vi "Topo & GridSpectr_DriftCorrection_v9.vi"(6 "Internal use":string, 7 "Grid param":T2 {"height (m)" format="%#_6p"; "width (m)" format="%#_6p"; "center Y (m)" format="%#_6p"; "center X (m)" format="%#_6p"}, 8 "Error in (no error)":errorcluster, 9 "Points Y/Index Y":i32, 10 "Points X/Index X":i32, 11 "Method":enum16{"init", "run", "end"}(ring)=enum."end") -> (0 "Error out":errorcluster)   [LabVIEW 2014]
doc: "Example of a measurement VI to be used in the \"Experiments on a Grid\" tool as external VI.\n\nThis example measure the topography and spectroscopy data. The spectroscopy measurements are taken on a subgrid. The data are saved to a sxm and a binary file.\n\n- Nanonis Programming Interface -"
uses:
  <userlib>/Nanonis Prog Interface V5/Nanonis Prog Interface.lvlib
  <userlib>/Nanonis Prog Interface V5/Scan/Grid/GridPatternGet.vi
panel:
  out "ETA":timestamp
  out "remaining":dbl
  out "Progress":u8(slide) scale=0.0..100.0 scale format="%#.1g"
  out "total Points":i32
  in  "preSTS delay [ms]":u32=3
  in  "STS Bias":dbl=0.005 format="%#_6p"
  in  "Move Bias":dbl=-0.01 format="%#_6p"
  in  "Move Current":dbl=1.5e-11 format="%#_6p"
  in  "Imaging Bias":dbl=-0.01 format="%#_6p"
  in  "max applied Drift Correction":i32=20 min=1 max=100 step=1 format="%.0p"
  in  "Correlate":u16(ring) items=["first Frame", "successive Frames"]
  out "Topo Images taken":i32=14
  in  "Increment":i32=40
  in  "Threshold":i32=2 min=1 step=1
  in  "tip Speed (m/s)":sgl=1e-08 format="%.2p"
  in  "Drift Correction 2":T1
  out "X drift":i32
  out "Y drift":i32
  out "Last Drift detected":i32=40
  in  "MaxImagesBack":i32=40
  in  "Channel index (0-23)":u8=14
  in  "File name":string="single_mol_shortSTS"
  in  "STS Current":dbl=1.15e-09 format="%#_6p"
  in  "Imaging Current":dbl=1.5e-11 format="%#_6p"
  in  "zdrift \nDuration (s)":dbl
  in  "Correct z drift":bool
  out "Status":string="finishing"
  in  "Drift correction Pixels":i32=256 caption="Topo Pixels"
  out "Y Offset":dbl format="%#_6p"
  out "X Offset":dbl format="%#_6p"
  out "Points taken":dbl=14.0
  in  "Drift Correction every":i32=40
  in  "Y subgrid spacing":u16=1
  in  "X subgrid spacing":u16=1
  # "GRID points"
  # "Increase this if no Drift was detected for \na certain number of images"
  # "images back"
  # "% of image size"
  # "RUN smart tilt before starting the GRID"
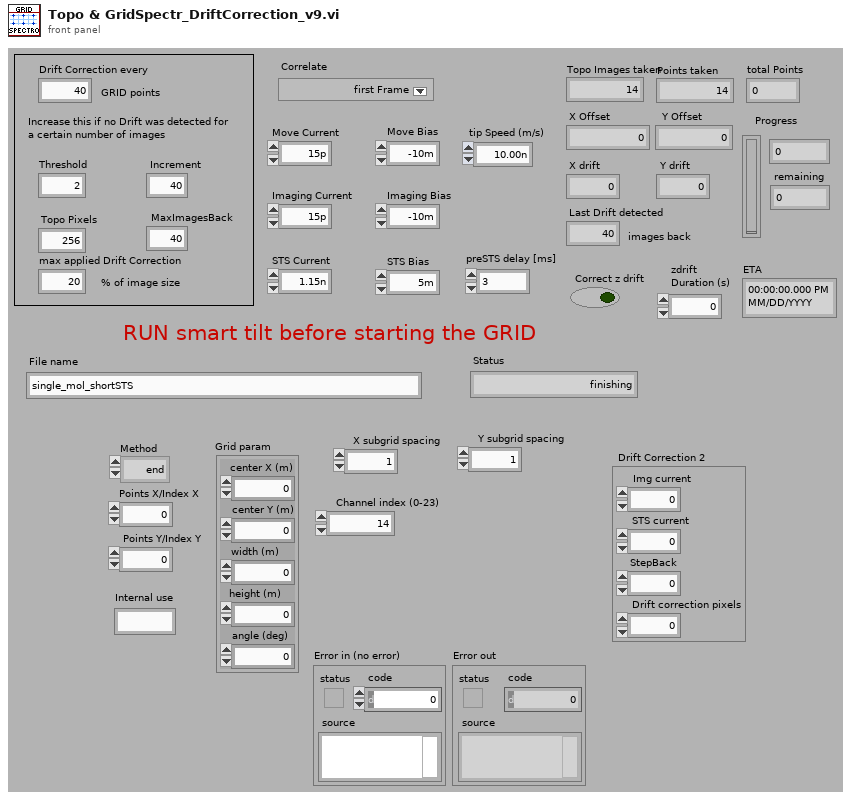
[diagram p1: front panel]
types:
  T1 = cluster{"Img current":dbl, "STS current":dbl, "StepBack":dbl, "Drift correction pixels":dbl}
  T2 = cluster{"center X (m)":sgl, "center Y (m)":sgl, "width (m)":sgl, "height (m)":sgl, "angle (deg)":sgl}
  T3 = cluster{"center X":sgl, "center Y":sgl, "angle":sgl, "width":sgl, "height":sgl, "# pixels":i32, "# lines":i32}
  T4 = cluster{"Name":string, "Calibration":sgl, "Offset":sgl, "Channel index":i32}[]
  T5 = cluster{"up/down":bool, "time/line":sgl, "start time":timestamp, "end time":timestamp}
  T6 = cluster{"Z averaging time (s)":sgl, "Z offset (m)":sgl, "Initial settling time (s)":sgl}
  T7 = cluster{"Max. slew rate (V/s)":sgl, "Settling time (s)":sgl, "Integration time (s)":sgl}
  T8 = cluster{"End settling time (s)":sgl, "Z control time (s)":sgl}
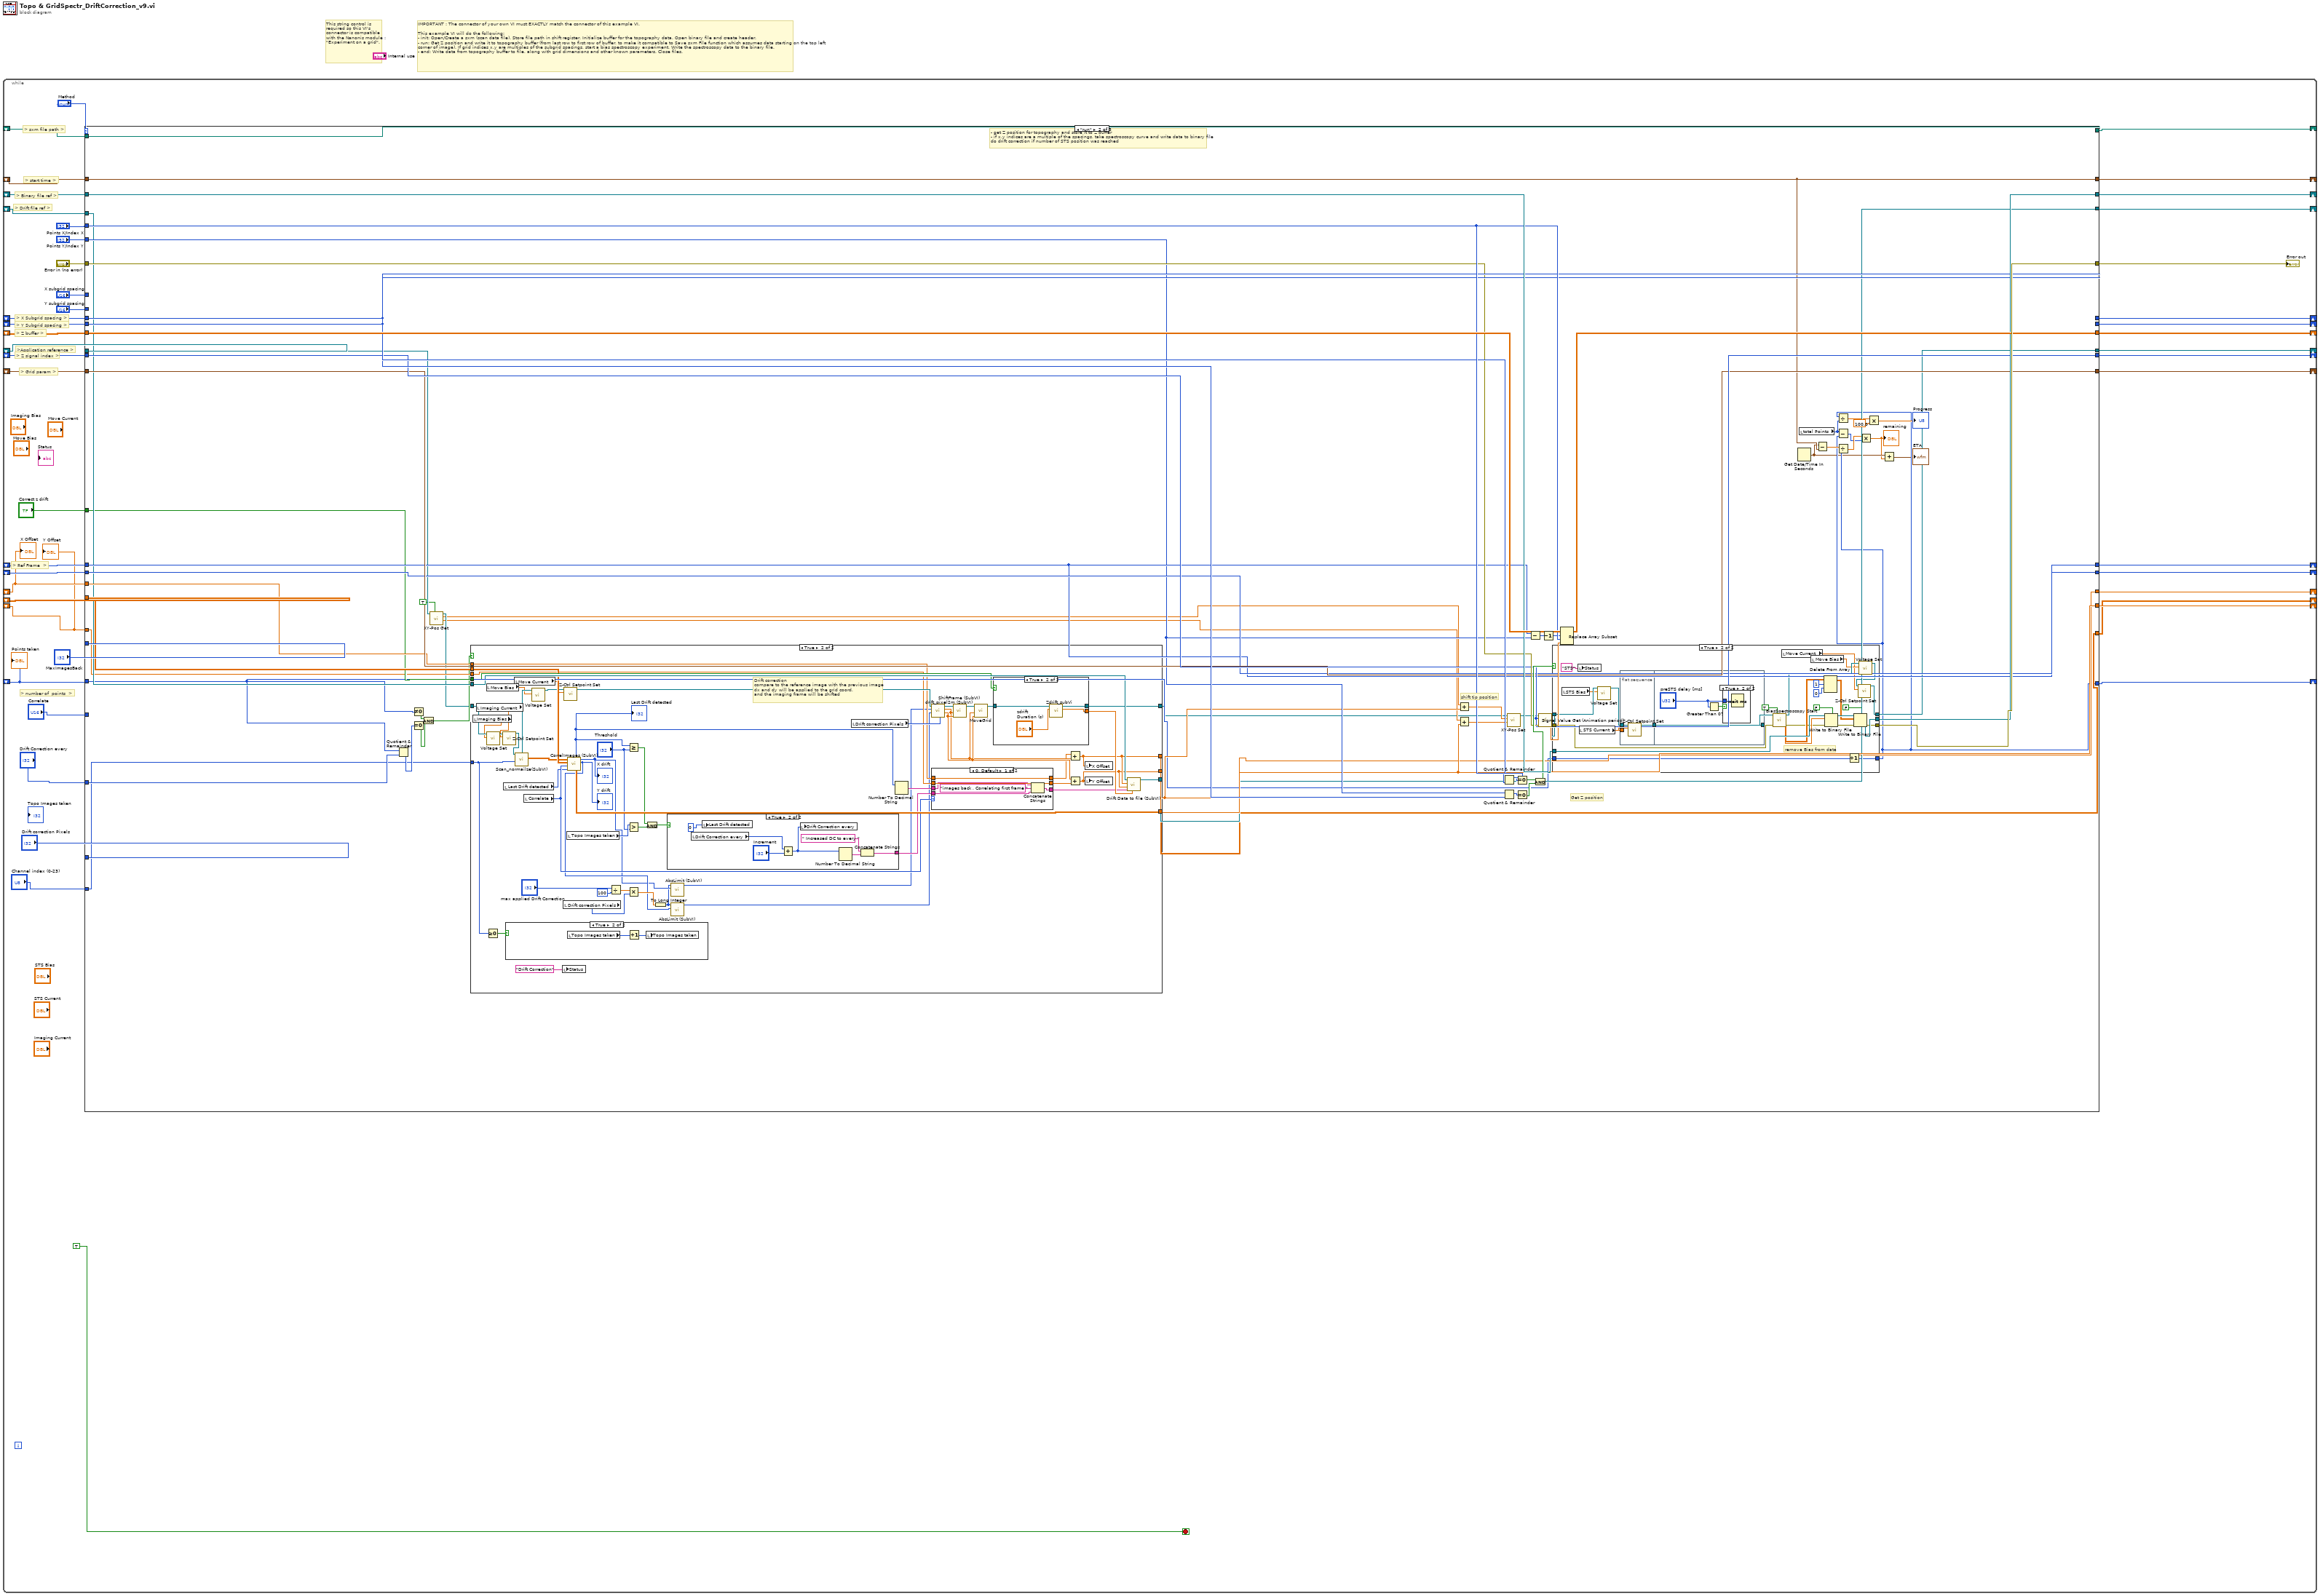
[diagram p0: block diagram]
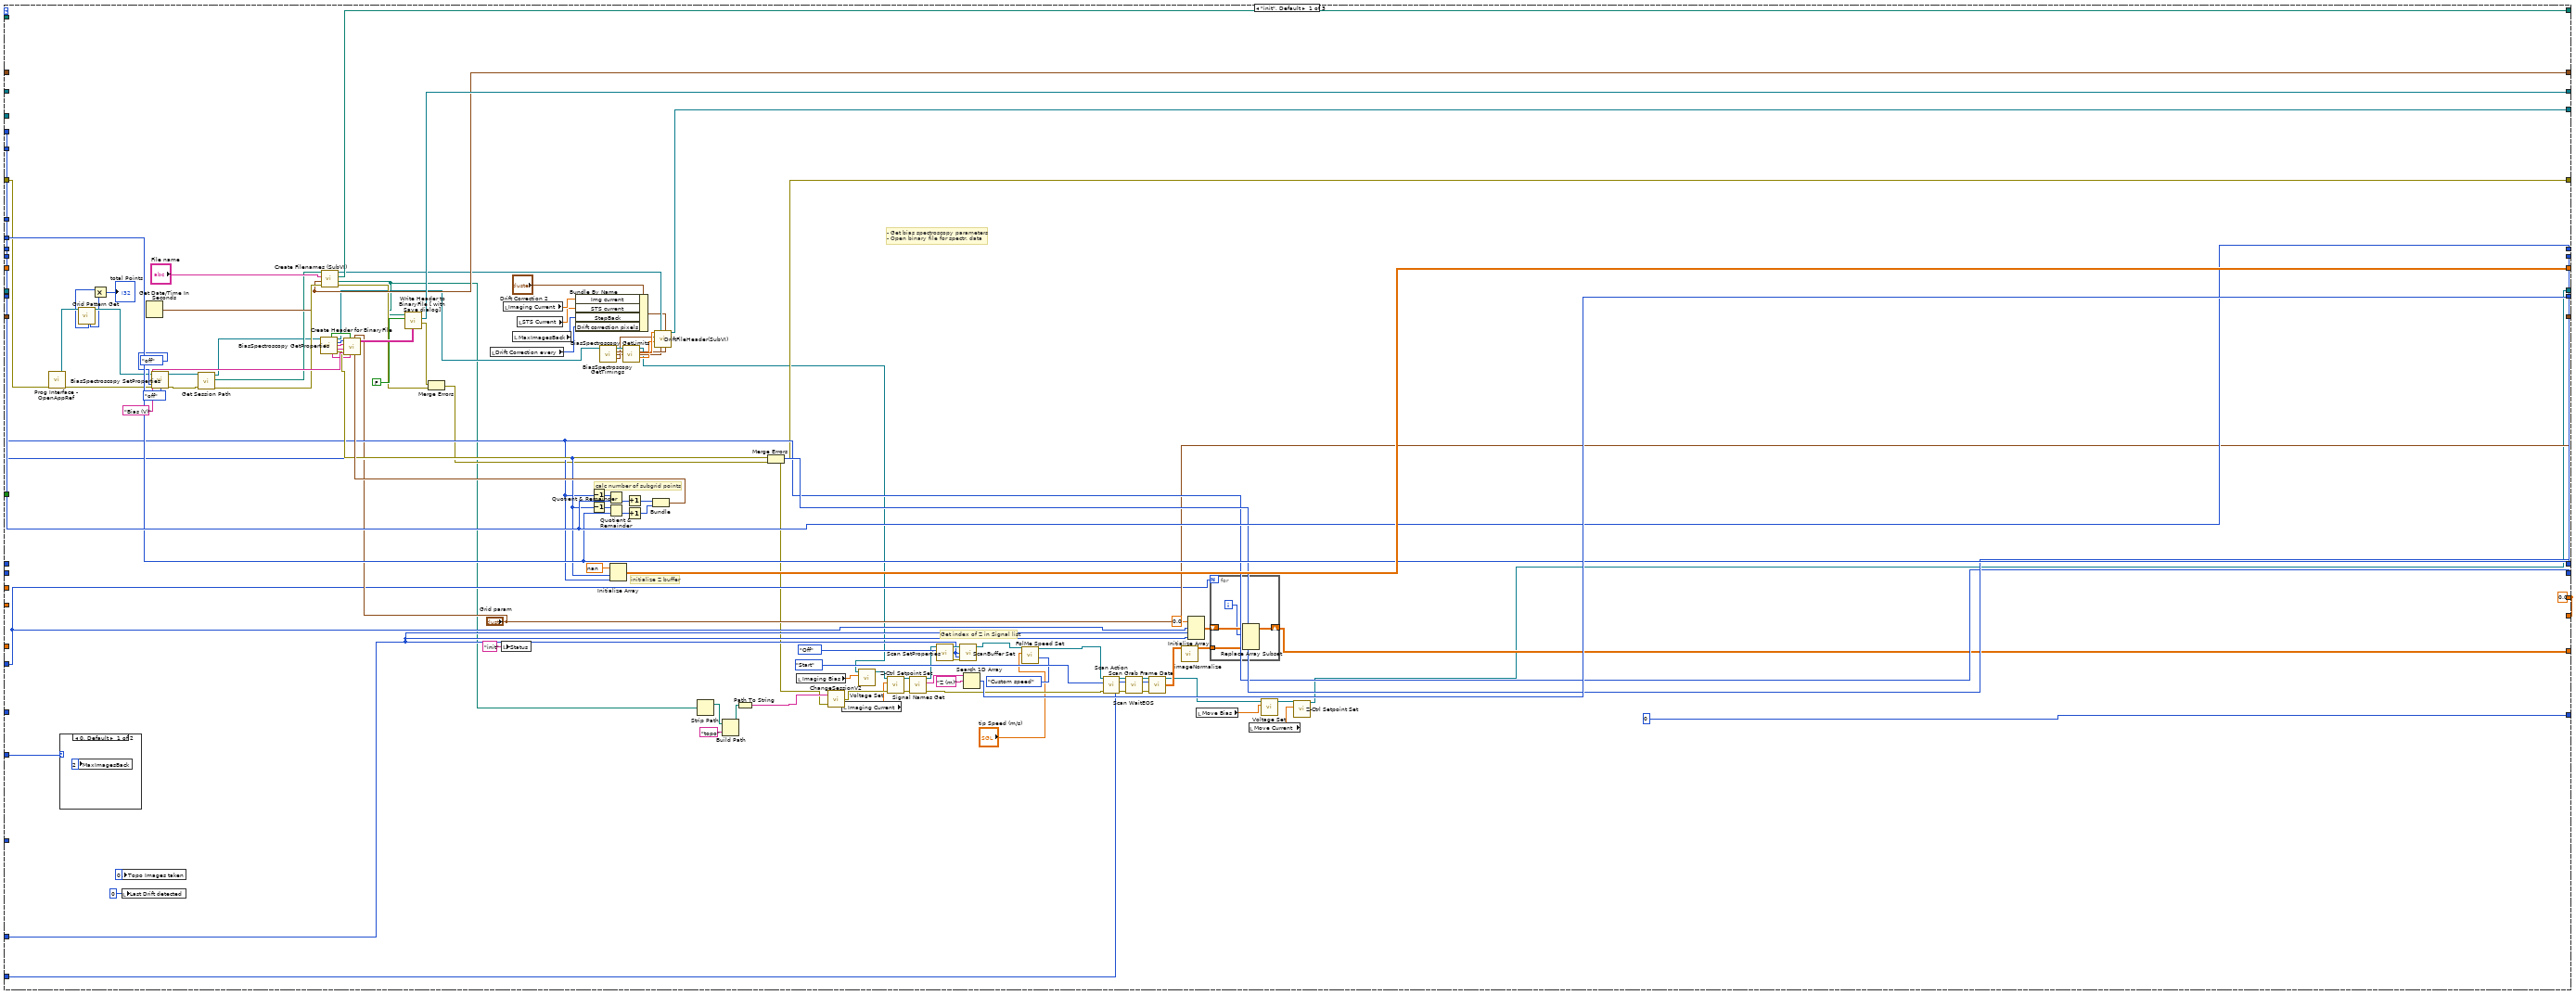
[diagram p2: hidden frame]
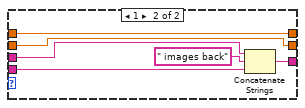
[diagram p5: hidden frame]
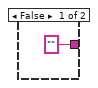
[diagram p7: hidden frame]
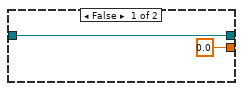
[diagram p8: hidden frame]
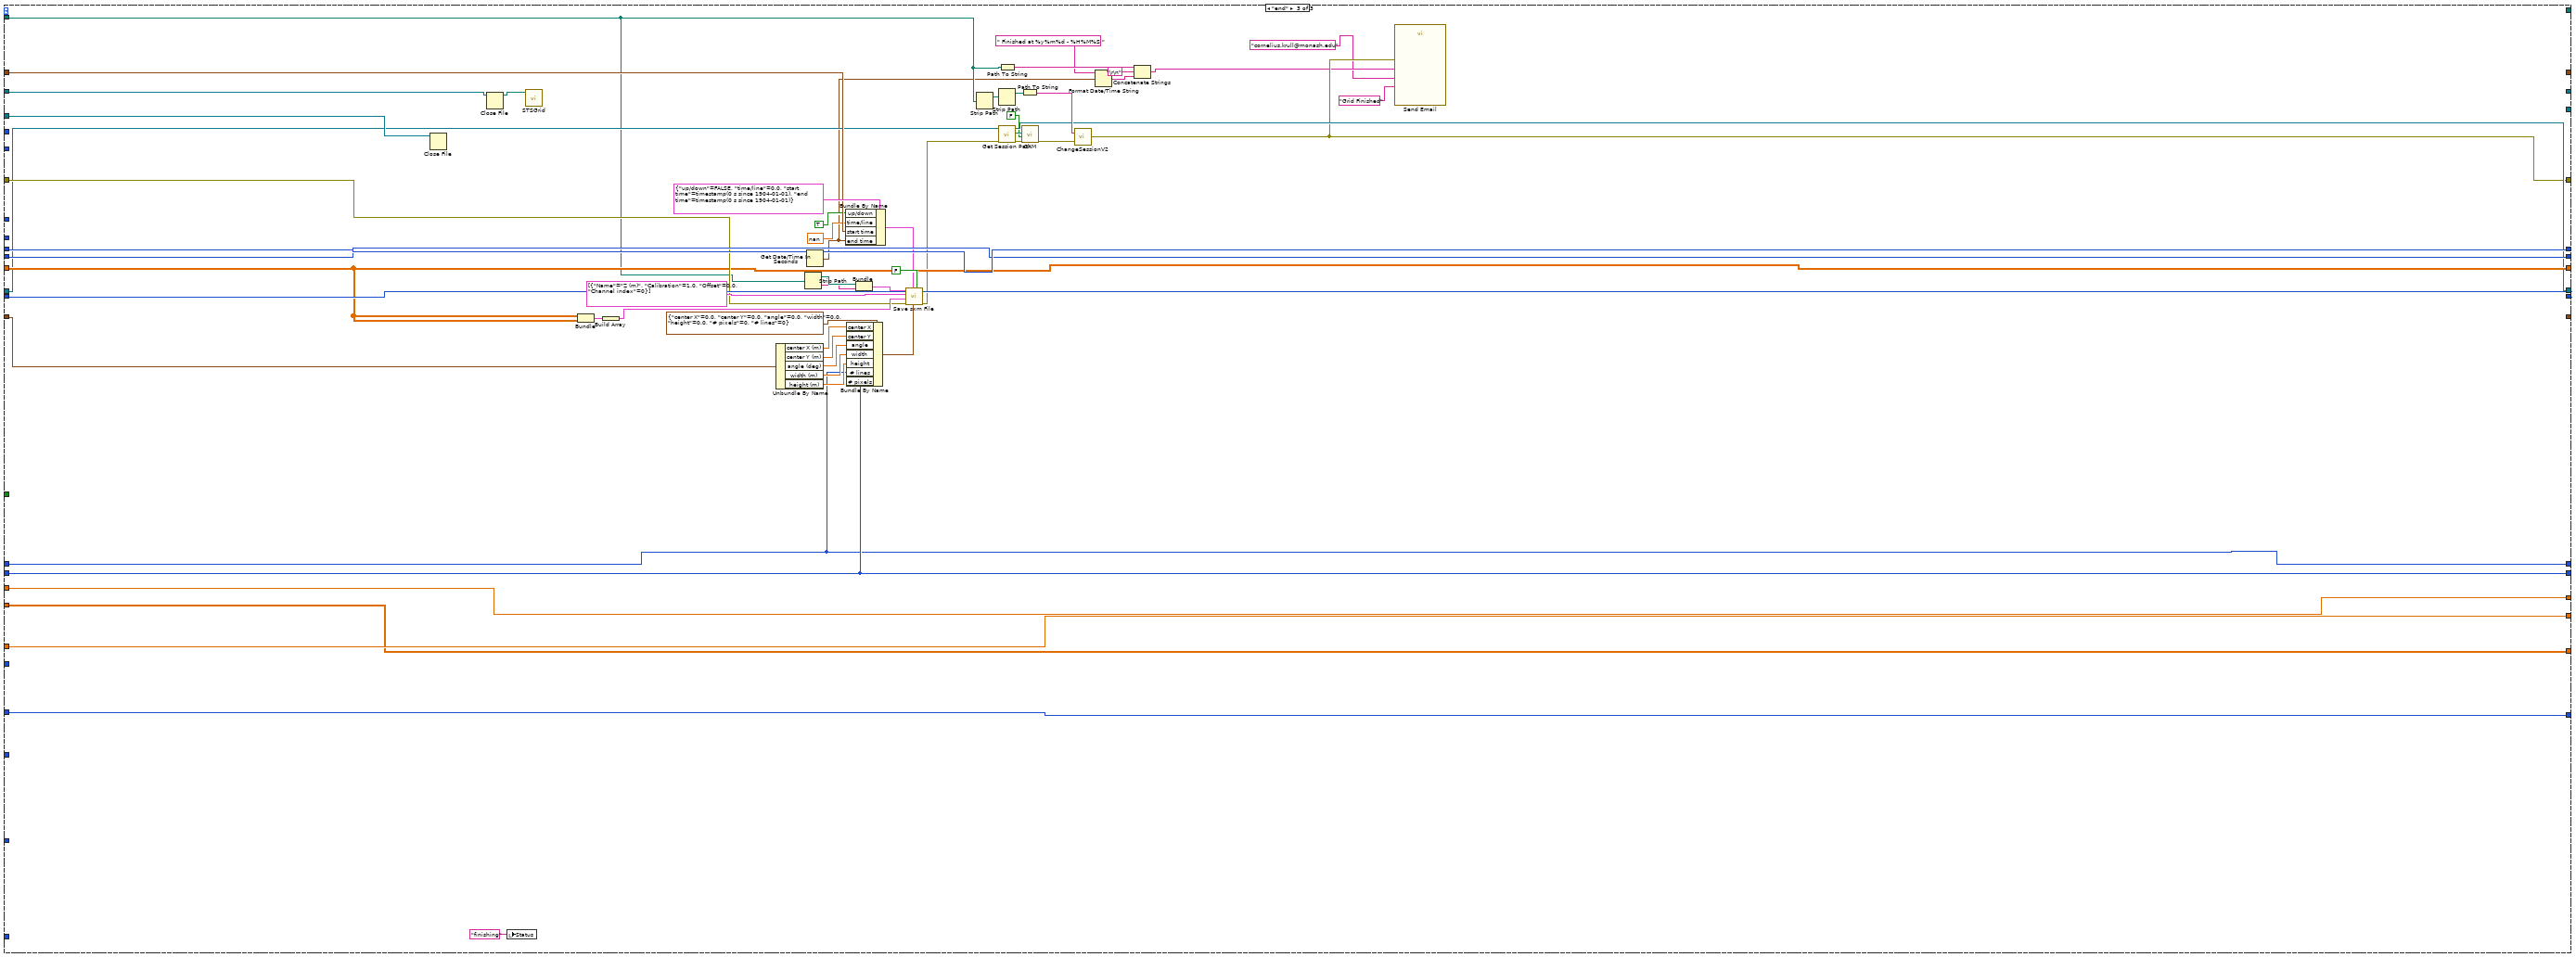
[diagram p11: hidden frame]
diagram:
  # "This string control is required so this VI's connector is compatible with the Nanonis module : \"Experiment on a grid\"."
  # "IMPORTANT : The connector of your own VI must EXACTLY match the connector of this example VI.\n\nThis example VI will do the following:\n- init: Open/Create a sxm (scan data file). Store file path in shift register. Initialize buffer for the topography data. Open binary file and create header.\n- run: Get Z position and write it to topography buffer (from last row to first row of buffer, to make it compatible to Save sxm File function which assumes data starting on the top left corner of image). If grid indices x,y are multiples of the subgrid spacings, start a bias spectroscopy experiment. Write the spectroscopy data to the binary file.\n- end: Write data from topography buffer to file, along with grid dimensions and other known parameters. Close files."
  n1 = while {
    shift-right: [w21] -> _
    shift-left: _ -> [w44]
    shift-right: [w39] -> _
    shift-left: _ -> [w38]
    shift-right: [w36] -> _
    shift-left: _ -> [w37]
    shift-right: [w35] -> _
    shift-left: _ -> [w34]
    shift-right: [w28] -> _
    shift-left: _ -> [w30]
    shift-right: [w29] -> _
    shift-left: _ -> [w31]
    shift-right: [w27] -> _
    shift-left: _ -> [w26]
    shift-right: [w25] -> _
    shift-left: _ -> [w24]
    shift-right: [w23] -> _
    shift-left: _ -> [w22]
    shift-right: [w20] -> _
    shift-left: _ -> [w19]
    shift-right: [w18] -> _
    shift-left: _ -> [w17]
    shift-right: [w16] -> _
    shift-left: _ -> [w9]
    shift-right: [w15] -> _
    shift-left: _ -> [w8]
    shift-right: [w14] -> _
    shift-left: _ -> [w11]
    shift-right: [w13] -> _
    shift-left: _ -> [w10]
    shift-right: [w6] -> _
    shift-left: _ -> [w5]
    stop <- TRUE stop-if-true
    # "> Drift file ref >"
    # "> number of  points  >"
    # "> Ref Frame  >"
    # "> Grid param >"
    # "> start time >"
    # ">Application reference >"
    # "> Y Subgrid spacing >"
    # "> X Subgrid spacing >"
    # "> Z signal index >"
    # "> Binary file ref >"
    # "> Z buffer >"
    # "> sxm file path >"
    n2 = case shown="\"run\"" "Method" {
      tunnel: [w109 w222 _] -> w21
      tunnel: w44 -> [_ w222 w358]
      tunnel: "Error in (no error)" -> [w111 w208 w390]
      tunnel: [w72 w221 w359] -> w42
      tunnel: "Points X/Index X" -> [w130 w216 _]
      tunnel: "Points Y/Index Y" -> [w131 w201 _]
      tunnel: [w154 w219 w379] -> w39
      tunnel: w38 -> [_ w220 w379]
      tunnel: w37 -> [_ w218 w372]
      tunnel: [w146 w217 _] -> w36
      tunnel: [w144 w206 w404] -> w35
      tunnel: w34 -> [_ w206 w404]
      tunnel: "X subgrid spacing" -> [w143 _ _]
      tunnel: "Y subgrid spacing" -> [w142 _ _]
      tunnel: w31 -> [_ w210 w403]
      tunnel: w30 -> [_ w209 w402]
      tunnel: [w143 w210 w403] -> w29
      tunnel: [w142 w209 w402] -> w28
      tunnel: [w60 w194 w364] -> w27
      tunnel: w26 -> [_ w177 w365]
      tunnel: ["Grid param" w204 _] -> w25
      tunnel: w24 -> [_ w204 w389]
      tunnel: [w108 w167 _] -> w23
      tunnel: w22 -> [_ w167 w397]
      tunnel: [w131 w202 w380] -> w20
      tunnel: w19 -> [_ w202 w380]
      tunnel: [w130 w203 w381] -> w18
      tunnel: w17 -> [_ w203 w381]
      tunnel: [w121 w184 w378] -> w16
      tunnel: [w121 w189 w376] -> w15
      tunnel: [w103 w183 w373] -> w14
      tunnel: [0 w165 w377] -> w13
      tunnel: w10 -> [_ w180 w377]
      tunnel: "Drift Correction every" -> [_ w197 _]
      tunnel: w11 -> [_ w188 w373]
      tunnel: w9 -> [_ w195 w378]
      tunnel: w8 -> [_ w181 w376]
      tunnel: "Drift correction Pixels" -> [w102 _ _]
      tunnel: [w98 w186 _] -> w6
      tunnel: w5 -> [_ w187 w374]
      tunnel: "Correct z drift" -> [_ w185 _]
      tunnel: "Channel index (0-23)" -> [w106 w182 _]
      tunnel: "MaxImagesBack" -> [w101 _ _]
      tunnel: "Correlate" -> [w63 _ _]
      frame "init", Default {
        w121 = 0.0
        # "- Get bias spectroscopy parameters\n- Open binary file for spectr. data"
        # "initialize Z buffer"
        # "calc number of subgrid points"
        # "Get index of Z in Signal list"
        n3 = call <userlib>:"Prog Interface - OpenAppRef.vi"("Error in (no error)"=w111) -> ("Error out"=w70:errorcluster, "Application reference"=w51:refnum<vi>)  [unwired: 5 in]
        n4 = case shown="0, Default" w63 {
          frame 0, Default {
            n5 = local write "MaxImagesBack"(2 ("StepsBack")) -> ()
          }
          frame 1 {
          }
        }
        n6 = call-poly <userlib>:"Grid Pattern Get.vi"("Application ref in"=w51) -> ("Points Y"=w48:i32, "Points X"=w49:i32, "Application ref out"=w50:refnum<vi>)  [unwired: 10 in, 6 out]
        n7 = Multiply(x=w48, y=w49) -> (x*y=→"total Points":i32)
        n8 = local write "Topo Images taken"(0 ("Images taken")) -> ()
        n9 = local write "Last Drift detected"(0 ("Last Drift detected")) -> ()
        n10 = Get Date/Time In Seconds() -> (seconds since 1Jan1904=w108:timestamp)
        n11 = call <userlib>:"BiasSpectroscopy SetProperties.vi"("Application ref in"=w50, "Autosave (no change)"=enum16{"no change", "on", "off"}."off", "Error in (no error)"=w70, "Save dialog"=enum16{"no change", "on", "off"}."off") -> ("Application ref out"=w66:refnum<vi>, "Error out"=w65:errorcluster)  [unwired: 10 in]
        n12 = call <userlib>:"Get Session Path.vi"("error in (no error)"=w65, "Application ref in"=w66) -> ("error out"=w110:errorcluster, "Session path"=w78:path, "Application ref out"=w67:refnum<vi>)  [unwired: 7 in]
        n13 = call <userlib>:"BiasSpectroscopy GetProperties.vi"("Application ref in"=w67) -> ("Backward sweep"=w150:bool, "Application ref out"=w82:refnum<vi>, "Number of points"=w133:i32, "Channels"=w132:string[], "Parameters"=w148:string[], "Fixed parameters"=w135:string[], "Error out"=w147:errorcluster)  [unwired: 6 in, 2 out]
        n14 = call "Create Filenames (SubVI).vi"("error in (no error)"=w110, "seconds since 1Jan1904"=w108, "File name"="File name", "Session path"=w78) -> ("error out"=w83:errorcluster, "binFilePath"=w74:path, "topoFilePath"=w109:path, "Drift File out"=w99:refnum<file>)  [unwired: 4 in]
        n15 = local read "Drift Correction every"() -> (w93:i32)
        n16 = local write "Status"("init" ("Status")) -> ()
        n17 = local read "Imaging Current"() -> (w95:dbl)
        n18 = local read "MaxImagesBack"() -> (w92:i32)
        n19 = local read "STS Current"() -> (w94:dbl)
        n20 = Bundle By Name(cluster="Drift Correction 2", "Img current"=w95, "STS current"=w94, "StepBack"=w92, "Drift correction pixels"=w93) -> (w96:T1)
        n21 = Decrement(x=w130) -> (x-1=w141:i32)
        n22 = Decrement(x=w131) -> (x-1=w140:i32)
        n23 = call <userlib>:"BiasSpectroscopy GetTimings.vi"("Application ref in"=w82) -> ("Application ref out"=w91:refnum<vi>, "Initialization"=w88:T6, "Sweep Timing"=w86:T7, "End of Sweep"=w87:T8)  [unwired: 10 in, 1 out]
        n24 = Quotient & Remainder(x=w141, y=w143) -> (floor(x/y)=w139:i32)  [unwired: 1 out]
        n25 = Quotient & Remainder(x=w140, y=w142) -> (floor(x/y)=w138:i32)  [unwired: 1 out]
        n26 = Initialize Array(sgl nan ("element"), w131, w130) -> (w154:sgl[][])
        n27 = call <userlib>:"BiasSpectroscopy GetLimits.vi"("Application ref in"=w91) -> ("End value (V)"=w89:sgl, "Start value (V)"=w90:sgl, "Application ref out"=w58:refnum<vi>)  [unwired: 5 in, 1 out]
        n28 = Increment(x=w139) -> (x+1=w137:i32)
        n29 = Increment(x=w138) -> (x+1=w136:i32)
        n30 = Bundle(w137, w136) -> (w149:cluster{i32, i32})  [unwired: 1 in]
        n31 = call <userlib>:"Create Header for BinaryFile.vi"("Grid points"=w149, "Grid param"="Grid param", "Fixed parameters"=w135, "Backward sweep"=w150, "Sweep signal"="Bias (V)" ("Sweep Signal"), "Parameters"=w148, "Channels"=w132, "Points per sweep"=w133) -> ("Header (fixed attributes)"=w152:string[][])  [unwired: 3 in]
        n32 = call <userlib>:"Write Header to BinaryFile [ with Save dialog].vi"("Fixed Attributes"=w152, "Show Dialog? (T)"=FALSE, "Filename"=w74) -> ("Error out"=w84:errorcluster, "File ref"=w146:refnum<file>)  [unwired: 5 in, 2 out]
        n33 = Merge Errors(w84, w83) -> (w85:errorcluster)
        n34 = call "DriftFileHeader(SubVI).vi"("Initialization"=w88, "Drift Correction"=w96, "Sweep Timing"=w86, "Byte Stream File in"=w99, "End value (V)"=w89, "End of Sweep"=w87, "Start value (V)"=w90) -> ("Byte Stream File out"=w98:refnum<file>)  [unwired: 4 in]
        n35 = Strip Path(path=w74) -> (stripped path=w77:path)  [unwired: 1 out]
        n36 = Build Path(base path=w77, name or relative path="topo") -> (appended path=w75:path)
        n37 = Path To String(path=w75) -> (string=w73:string)
        n38 = Merge Errors(w147, w85) -> (w72:errorcluster)
        n39 = local read "Imaging Bias"() -> (w54:dbl)
        n40 = call "ChangeSessionV2.vi"("error in (no error)"=w72, "Session"=w73) -> ("error out"=w71:errorcluster)
        n41 = local read "Imaging Current"() -> (w53:dbl)
        n42 = call <userlib>:"Voltage Set.vi"("Bias (V)"=w54, "Application ref in"=w58) -> ("Application ref out"=w57:refnum<vi>)  [unwired: 8 in, 1 out]
        n43 = call <userlib>:"Z-Ctrl Setpoint Set.vi"("error in (no error)"=w71, "Z Controller setpoint"=w53, "Application ref in"=w57) -> ("error out"=w112:errorcluster, "Application ref out"=w113:refnum<vi>)  [unwired: 7 in]
        n44 = call <userlib>:"Signal Names Get.vi"("error in (no error)"=w112, "Application ref in"=w113) -> ("error out"=w122:errorcluster, "Signals Names"=w134:string[], "Application ref out"=w117:refnum<vi>)  [unwired: 5 in]
        n45 = call <userlib>:"Scan SetProperties.vi"("Application ref in"=w117, "Continuous scan"=enum16{"No change", "On", "Off"}."Off") -> ("Application ref out"=w119:refnum<vi>, "Error out"=w118:errorcluster)  [unwired: 12 in]
        n46 = call <userlib>:"ScanBuffer Set.vi"("Application ref in"=w119, "Pixels"=w102, "Lines"=w102, "error in (no error)"=w118) -> ("Application ref out"=w61:refnum<vi>)  [unwired: 10 in, 1 out]
        n47 = Search 1D Array(1D array=w134, element="Z (m)") -> (index of element=w144:i32)  [unwired: 1 in]
        n48 = call <userlib>:"FolMe Speed Set.vi"("Speed Setting (Custom)"=enum32{"Scan speed", "Custom speed"}."Custom speed", "Speed (m/s)"="tip Speed (m/s)", "Application ref in"=w61) -> ("Application ref out"=w81:refnum<vi>)  [unwired: 5 in, 1 out]
        n49 = call <userlib>:"Scan Action.vi"("error in (no error)"=w122, "Scan action (Start)"=enum16{"Start", "Stop", "Pause", "Resume"}."Start", "Application ref in"=w81) -> ("error out"=w128:errorcluster, "Application ref out"=w127:refnum<vi>)  [unwired: 6 in]
        n50 = call <userlib>:"Scan WaitEOS.vi"("error in (no error)"=w128, "Application ref in"=w127) -> ("error out"=w125:errorcluster, "Application ref out"=w126:refnum<vi>)  [unwired: 5 in, 2 out]
        n51 = call <userlib>:"Scan Grab Frame Data.vi"("Application ref in"=w126, "Channel index (0-23)"=w106, "error in (no error)"=w125) -> ("Application ref out"=w52:refnum<vi>, "Scan frame data"=w114:sgl[][])  [unwired: 8 in, 3 out]
        n52 = call "imageNormalize.vi"("Data"=w114) -> ("Array"=w100:dbl[][])  [unwired: 10 in]
        n53 = Initialize Array(0.0 ("element"), w101, w102, w102) -> (w104:dbl[][][])
        n54 = local read "Move Bias"() -> (w56:dbl)
        n55 = for {
          N: w101 -> [_]
          tunnel: w100 -> [w158]
          shift-right: [w157] -> w103
          shift-left: w104 -> [w159]
          i -> [w156]
          n56 = Replace Array Subset(array=w159, new element=w158, index (dim 0)=w156) -> (w157:dbl[][][])  [unwired: 2 in]
        }
        n57 = local read "Move Current"() -> (w55:dbl)
        n58 = call <userlib>:"Voltage Set.vi"("Bias (V)"=w56, "Application ref in"=w52) -> ("Application ref out"=w59:refnum<vi>)  [unwired: 8 in, 1 out]
        n59 = call <userlib>:"Z-Ctrl Setpoint Set.vi"("Z Controller setpoint"=w55, "Application ref in"=w59) -> ("Application ref out"=w60:refnum<vi>)  [unwired: 8 in, 1 out]
      }
      frame "run" {
        # "shift tip position"
        # "Get Z position"
        # "- get Z position for topography and store it to Z buffer\n- if x,y indices are a multiple of the spacings, take spectroscopy curve and write data to binary file\ndo drift correction if number of STS position was reached"
        n60 = Quotient & Remainder(x=w180, y=w197) -> (x-y*floor(x/y)=w198:i32)  [unwired: 1 out]
        n61 = Not Equal To 0?(x=w180) -> (x != 0?=w178:bool)
        n62 = Equal To 0?(x=w198) -> (x = 0?=w196:bool)
        n63 = And(x=w178, y=w196) -> (x .and. y?=w179:bool)
        n64 = call <userlib>:"XY-Pos Get.vi"("Wait for newest data (F=False)"=TRUE, "Application ref in"=w177) -> ("Y (m)"=w173:sgl, "X (m)"=w174:sgl, "Application ref out"=w176:refnum<vi>)  [unwired: 5 in, 1 out]
        n65 = case shown="True" w179 {
          tunnel: w176 -> [w227 w235]
          tunnel: [w227 w277] -> w172
          tunnel: w188 -> [w224 w272]
          tunnel: [w226 w275] -> w184
          tunnel: [w225 w274] -> w189
          tunnel: w195 -> [w226 w251]
          tunnel: w181 -> [w225 w249]
          tunnel: [w224 w268] -> w183
          tunnel: w187 -> [w223 w280]
          tunnel: [w223 w279] -> w186
          tunnel: w185 -> [_ w276]
          tunnel: w182 -> [_ w255]
          frame False {
          }
          frame True {
            # "Drift correction \ncompare to the reference image with the previous image \ndx and dy will be applied to the grid coord, \nand the imaging frame will be shifted"
            n66 = local read "Imaging Bias"() -> (w233:dbl)
            n67 = local read "Imaging Current"() -> (w232:dbl)
            n68 = local read "Move Bias"() -> (w229:dbl)
            n69 = Greater Or Equal To 0?(x=w255) -> (x >= 0?=w254:bool)
            n70 = call <userlib>:"Voltage Set.vi"("Bias (V)"=w233, "Application ref in"=w235) -> ("Application ref out"=w234:refnum<vi>)  [unwired: 8 in, 1 out]
            n71 = call <userlib>:"Z-Ctrl Setpoint Set.vi"("Z Controller setpoint"=w232, "Application ref in"=w234) -> ("Application ref out"=w273:refnum<vi>)  [unwired: 8 in, 1 out]
            n72 = local read "Last Drift detected"() -> (w246:i32)
            n73 = case shown="True" w254 {
              frame False {
              }
              frame True {
                n74 = local read "Topo Images taken"() -> (w295:i32)
                n75 = Increment(x=w295) -> (x+1=w294:i32)
                n76 = local write "Topo Images taken"(w294) -> ()
              }
            }
            n77 = local read "Move Current"() -> (w228:dbl)
            n78 = call "Scan_normailze(SubVI).vi"("Channel index (0-23)"=w255, "Application in"=w273) -> ("Array"=w269:dbl[][], "Application out"=w230:refnum<vi>)  [unwired: 7 in, 1 out]
            n79 = local read "Correlate"() -> (w252:u16)
            n80 = call <userlib>:"Voltage Set.vi"("Bias (V)"=w229, "Application ref in"=w230) -> ("Application ref out"=w231:refnum<vi>)  [unwired: 8 in, 1 out]
            n81 = local write "Status"("Drift Correction" ("Status")) -> ()
            n82 = local read "Drift correction Pixels"() -> (w243:i32)
            n83 = call <userlib>:"Z-Ctrl Setpoint Set.vi"("Z Controller setpoint"=w228, "Application ref in"=w231) -> ("Application ref out"=w264:refnum<vi>)  [unwired: 8 in, 1 out]
            n84 = local read "Topo Images taken"() -> (w257:i32)
            n85 = call "CorrelImages (SubVI).vi"("last drift detected"=w246, "Correlate"=w252, "Ref Array"=w272, "New Image"=w269) -> ("Y drift"=w240:i32, "X drift"=w237:i32, "Ref Array out"=w268:dbl[][][], "Queue Steps"=w253:i32)  [unwired: 4 in]
            "X drift" <- w237
            "Y drift" <- w240
            "Last Drift detected" <- w253
            n86 = Divide(x="max applied Drift Correction", y=100) -> (x/y=w242:dbl)
            n87 = Greater Or Equal?(x=w253, y="Threshold") -> (x >= y?=w259:bool)
            n88 = Greater?(x=w257, y="Threshold") -> (0:w256:bool)
            n89 = Multiply(x=w242, y=w243) -> (x*y=w244:dbl)
            n90 = And(x=w259, y=w256) -> (x .and. y?=w258:bool)
            n91 = To Long Integer(number=w244) -> (32bit integer=w236:i32)
            n92 = case shown="True" w258 {
              tunnel: ["" w299] -> w260
              frame False {
              }
              frame True {
                n93 = local read "Drift Correction every"() -> (w298:i32)
                n94 = local write "Last Drift detected"(0 ("Last Drift detected")) -> ()
                n95 = Add(x=w298, y="Increment") -> (x+y=w302:i32)
                n96 = local write "Drift Correction every"(w302) -> ()
                n97 = Number To Decimal String(number=w302) -> (decimal integer string=w301:string)  [unwired: 1 in]
                n98 = Concatenate Strings(" Increased DC to every " ("string"), w301) -> (w299:string)
              }
            }
            n99 = call "AbsLimit (SubVI).vi"("in"=w237, "Abslimt"=w236) -> ("Numeric out"=w239:i32)  [unwired: 9 in]
            n100 = call "AbsLimit (SubVI).vi"("in"=w240, "Abslimt"=w236) -> ("Numeric out"=w238:i32)  [unwired: 9 in]
            n101 = local read "Drift correction Pixels"() -> (w265:i32)
            n102 = Number To Decimal String(number=w253) -> (decimal integer string=w271:string)  [unwired: 1 in]
            n103 = call "drift_pixel2m (SubVI).vi"("Application in"=w264, "X drift"=w239, "Y drift"=w238, "Drift correction Pixels"=w265) -> ("Application out"=w263:refnum<vi>, "x drift"=w261:sgl, "y drift"=w262:sgl)  [unwired: 2 in, 1 out]
            n104 = case shown="0, Default" w252 {
              tunnel: w271 -> [w282 w293]
              tunnel: [w287 w292] -> w270
              tunnel: w260 -> [w285 w290]
              tunnel: w251 -> [w283 w289]
              tunnel: [w283 w289] -> w250
              tunnel: w249 -> [w284 w288]
              tunnel: [w284 w288] -> w248
              frame 0, Default {
                n105 = Concatenate Strings(w282, "images back , Correlating first frame " ("string"), w285) -> (w287:string)
              }
              frame 1 {
                n106 = Concatenate Strings(w293, " images back" ("string"), w290) -> (w292:string)
              }
            }
            n107 = call "ShiftFrame (SubVI).vi"("Y shift"=w262, "X shift"=w261, "Application in"=w263) -> ("Application out"=w267:refnum<vi>)  [unwired: 8 in]
            n108 = call "MoveGrid.vi"("y"=w262, "x"=w261, "Application ref in"=w267) -> ("Application ref out"=w266:refnum<vi>)  [unwired: 7 in, 1 out]
            n109 = case shown="True" w276 {
              tunnel: [0.0 ("z drift") w309] -> w278
              tunnel: w266 -> [w304 w308]
              tunnel: [w304 w307] -> w277
              frame False {
              }
              frame True {
                n110 = call "Zdrift_subVi.vi"("Duration"="zdrift \nDuration (s)", "Application in"=w308) -> ("z drift"=w309:dbl, "Application out"=w307:refnum<vi>)  [unwired: 7 in, 1 out]
              }
            }
            n111 = Add(x=w250, y=w261) -> (x+y=w275:dbl)
            n112 = Add(x=w262, y=w248) -> (x+y=w274:dbl)
            n113 = local write "X Offset"(w275) -> ()
            n114 = local write "Y Offset"(w274) -> ()
            n115 = call "Drift Data to file (SubVI).vi"("z drift"=w278, "Comment"=w270, "y Drift"=w274, "X drift"=w275, "Byte Stream File in"=w280) -> ("Byte Stream File out"=w279:refnum<file>)  [unwired: 6 in]
          }
        }
        n116 = Add(x=w174, y=w184) -> (x+y=w191:dbl)
        n117 = Add(x=w173, y=w189) -> (x+y=w190:dbl)
        n118 = Quotient & Remainder(x=w216, y=w210) -> (x-y*floor(x/y)=w215:i32)  [unwired: 1 out]
        n119 = Quotient & Remainder(x=w201, y=w209) -> (x-y*floor(x/y)=w214:i32)  [unwired: 1 out]
        n120 = call <userlib>:"XY-Pos Set.vi"("Y (m)"=w190, "X (m)"=w191, "Application ref in"=w172) -> ("Application ref out"=w192:refnum<vi>)  [unwired: 5 in, 1 out]
        n121 = Equal To 0?(x=w215) -> (x = 0?=w213:bool)
        n122 = Equal To 0?(x=w214) -> (x = 0?=w212:bool)
        n123 = Subtract(x=w202, y=w201) -> (x-y=w200:i32)
        n124 = And(x=w213, y=w212) -> (x .and. y?=w211:bool)
        n125 = call <userlib>:"Signal Value Get (Animation period).vi"("error in (no error)"=w208, "Signal index (0-47)"=w206, "Application ref in"=w192) -> ("error out"=w207:errorcluster, "Signal value"=w205:sgl, "Application ref out"=w193:refnum<vi>)  [unwired: 5 in]
        n126 = Decrement(x=w200) -> (x-1=w199:i32)
        n127 = case shown="True" w211 {
          tunnel: [w312 w328] -> w221
          tunnel: w218 -> [w313 w342]
          tunnel: [w313 w340] -> w217
          tunnel: w207 -> [w312 w339]
          tunnel: w193 -> [w311 w324]
          tunnel: [w311 w316] -> w194
          tunnel: [w310 w326] -> w165
          tunnel: w180 -> [w310 w327]
          frame False {
            # "Point indices aren't multiple of subgrid spacing\n=> no spectroscopy at this point"
          }
          frame True {
            # "remove Bias from data"
            n128 = local read "STS Bias"() -> (w321:dbl)
            n129 = local write "Status"("STS" ("Status")) -> ()
            n130 = local read "STS Current"() -> (w320:dbl)
            n131 = call <userlib>:"Voltage Set.vi"("Bias (V)"=w321, "Application ref in"=w324) -> ("Application ref out"=w323:refnum<vi>)  [unwired: 8 in, 1 out]
            n132 = flat-sequence {
              tunnel: w323 -> [w345]
              tunnel: w320 -> [w343]
              tunnel: [w344] -> w319
              tunnel: [w348] -> w322
              tunnel: w319 -> [w348]
              frame #0 {
                n133 = call <userlib>:"Z-Ctrl Setpoint Set.vi"("Z Controller setpoint"=w343, "Application ref in"=w345) -> ("Application ref out"=w344:refnum<vi>)  [unwired: 8 in, 1 out]
              }
              frame #1 {
                n134 = Greater Than 0?(x="preSTS delay [ms]") -> (x > 0?=w346:bool)
                n135 = case shown="True" w346 {
                  tunnel: "preSTS delay [ms]" -> [_ w349]
                  frame False {
                  }
                  frame True {
                    n136 = Wait (ms)(milliseconds to wait=w349) -> ()  [unwired: 1 out]
                  }
                }
              }
            }
            n137 = call <userlib>:"BiasSpectroscopy Start.vi"("Application ref in"=w322, "Get data (F)"=TRUE ("Get Data (F)"), "Error in (no error)"=w339) -> ("Application ref out"=w318:refnum<vi>, "Data"=w338:sgl[][], "Parameters"=w337:sgl[], "Error out"=w330:errorcluster)  [unwired: 8 in, 1 out]
            n138 = local read "Move Current"() -> (w314:dbl)
            n139 = local read "Move Bias"() -> (w315:dbl)
            n140 = Delete From Array(array=w338, length=1, index (row)=0 ("index")) -> (array with subset deleted=w336:sgl[][])  [unwired: 1 in, 1 out]
            n141 = Write to Binary File(file (use dialog)=w342, data=w337, error in=w330, 5:FALSE ("prepend array or string size? (T)")) -> (refnum out=w341:refnum<file>, error out=w329:errorcluster)  [unwired: 2 in, 1 out]
            n142 = Increment(x=w327) -> (x+1=w326:i32)
            n143 = Write to Binary File(file (use dialog)=w341, data=w336, error in=w329, 5:FALSE ("prepend array or string size? (T)")) -> (refnum out=w340:refnum<file>, error out=w328:errorcluster)  [unwired: 2 in, 1 out]
            n144 = call <userlib>:"Voltage Set.vi"("Bias (V)"=w315, "Application ref in"=w318) -> ("Application ref out"=w317:refnum<vi>)  [unwired: 8 in, 1 out]
            n145 = call <userlib>:"Z-Ctrl Setpoint Set.vi"("Z Controller setpoint"=w314, "Application ref in"=w317) -> ("Application ref out"=w316:refnum<vi>)  [unwired: 8 in, 1 out]
          }
        }
        n146 = Replace Array Subset(array=w220, new element=w205, index (row)=w199, index (col)=w216) -> (w219:sgl[][])
        n147 = Get Date/Time In Seconds() -> (seconds since 1Jan1904=w162:timestamp)
        n148 = local read "total Points"() -> (w168:i32)
        n149 = Subtract(x=w162, y=w167) -> (x-y=w166:dbl)
        n150 = Divide(x=w165, y=w168) -> (x/y=w171:dbl)
        n151 = Subtract(x=w168, y=w165) -> (x-y=w163:i32)
        n152 = Divide(x=w166, y=w165) -> (x/y=w164:dbl)
        n153 = Multiply(x=w164, y=w163) -> (x*y=w161:dbl)
        "remaining" <- w161
        n154 = Multiply(x=w171, y=100.0) -> (x*y=→"Progress":dbl)
        n155 = Add(x=w162, y=w161) -> (x+y=→"ETA":timestamp)
      }
      frame "end" {
        n156 = Close File(refnum=w374) -> ()  [unwired: 1 in, 2 out]
        n157 = Close File(refnum=w372) -> (path=w371:path)  [unwired: 1 in, 1 out]
        n158 = local write "Status"("finishing" ("Status")) -> ()
        n159 = call "STSGrid.vi"("Binary Spectroscopy File"=w371) -> ()  [unwired: 11 in]
        n160 = Bundle(w379, w379) -> (w401:cluster{sgl[][], sgl[][]})  [unwired: 1 in]
        n161 = Build Array(w401) -> (w400:cluster{sgl[][], sgl[][]}[])
        n162 = Unbundle By Name(w389) -> ("center X (m)"=w387:sgl, "center Y (m)"=w386:sgl, "angle (deg)"=w385:sgl, "width (m)"=w384:sgl, "height (m)"=w383:sgl)
        n163 = Strip Path(path=w358) -> (stripped path=w393:path, name=w392:string)
        n164 = Get Date/Time In Seconds() -> (seconds since 1Jan1904=w353:timestamp)
        n165 = Bundle By Name(cluster=T5 {"up/down"=FALSE, "time/line"=0.0, "start time"=timestamp(0 s since 1904-01-01), "end time"=timestamp(0 s since 1904-01-01)} ("Scan param"), "up/down"=TRUE, "time/line"=sgl nan ("input 7"), "start time"=w397, "end time"=w353) -> (w396:T5)
        n166 = Bundle By Name(cluster=T3 {"center X"=0.0, "center Y"=0.0, "angle"=0.0, "width"=0.0, "height"=0.0, "# pixels"=0, "# lines"=0} ("Scanfield"), "center X"=w387, "center Y"=w386, "angle"=w385, "width"=w384, "height"=w383, "# lines"=w380, "# pixels"=w381) -> (w382:T3)
        n167 = Bundle("stripped path"=w393, "name"=w392) -> (w391:cluster{"stripped path":path, "name":string})  [unwired: 1 in]
        n168 = call <userlib>:"Save sxm File.vi"("Auto file naming? (T)"=FALSE, "Scanfield"=w382, "Scan param"=w396, "error in (no error)"=w390, "Channels data"=w400, "Channels config"=T4 [{"Name"="Z (m)", "Calibration"=1.0, "Offset"=0.0, "Channel index"=0}], "Filename control"=w391) -> ("error out"=w366:errorcluster)  [unwired: 2 in, 2 out]
        n169 = Strip Path(path=w358) -> (stripped path=w370:path)  [unwired: 1 out]
        n170 = Strip Path(path=w370) -> (stripped path=w369:path)  [unwired: 1 out]
        n171 = call <userlib>:"Get Session Path.vi"("error in (no error)"=w366, "Application ref in"=w365) -> ("error out"=w361:errorcluster, "Session path"=w363:path, "Application ref out"=w364:refnum<vi>)  [unwired: 7 in]
        n172 = Path To String(path=w358) -> (string=w357:string)
        n173 = Path To String(path=w369) -> (string=w367:string)
        n174 = call "SXM.vi"("Path"=w363, "Delete"=FALSE, "error in"=w361) -> ("error out"=w360:errorcluster)  [unwired: 7 in]
        n175 = call "ChangeSessionV2.vi"("error in (no error)"=w360, "Session"=w367) -> ("error out"=w359:errorcluster)
        n176 = Format Date/Time String(time format string (%c)=" Finished at %y%m%d - %H%M%S ", seconds (now)=w353) -> (date/time string=w352:string)  [unwired: 1 in]
        n177 = Concatenate Strings(w357, "\r\n", w352) -> (w355:string)
        n178 = call "Send Email"("error in"=w359, "Message"=w355, "Subject"="Grid Finished", "Recipients"="cornelius.krull@monash.edu") -> ()  [unwired: 7 in, 1 out]
      }
    }
    "Error out" <- w42
    "Points taken" <- w10
    "X Offset" <- w9
    "Y Offset" <- w8
  }
